vi "PCO_GetStorageStruct.vi"(8 "error in (no error)":errorcluster {"code" format="%x"}, 11 "ph":u64) -> (0 "error out":errorcluster {"code" format="%x"}, 1 "strStorage":T1, 2 "ErrorMessage":i32 format="%x", 3 "ph out":u64)   [LabVIEW 2019, in "SDK.lvlib" / "StorageControl.lvlib"]
doc: "<b>Description:</b>\nInformation about camera internal memory (CamRAM) is queried from the camera and the variables of the PCO_Storage structure are filled with this information. This function is a combined version of the functions, which request information about the current settings of storage related parameter. For a detailed description of each parameter see the functions in this chapter.\n\n<b>Supported camera type:</b>\npco.dimax, pco.1200, pco.1600, pco.2000, pco.4000\n\n<b>Descriptor dependency:</b>\ndwGeneralCapsDESC1: NO_RECORDER"
uses:
  StorageControl.lvlib
  Structures/Structures.lvlib
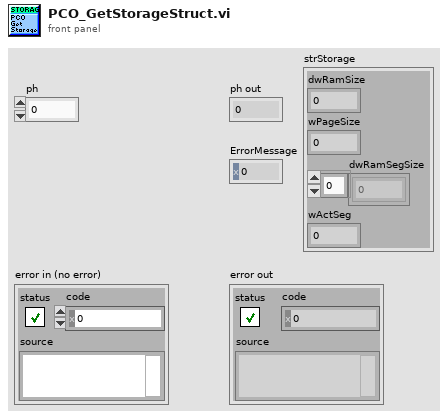
[diagram p1: front panel]
types:
  T1 = cluster{"dwRamSize":u32, "wPageSize":u16, "dwRamSegSize":u32[], "wActSeg":u16}
  T2 = cluster{"wSize":u16, "ZZwAlignDummy1":u16, "dwRamSize":u32, "wPageSize":u16, "ZZwAlignDummy4":u16, "dwRamSegSize":cluster{u32, u32, u32, u32}, "ZZdwDummyrs":cluster{u32, u32, u32, u32, u32, u32, u32, u32, u32, u32, u32, u32, u32, u32, u32, u32, u32, u32, u32, u32}, "wActSeg":u16, "ZZwDummy":cluster{u16, u16, u16, u16, u16, u16, u16, u16, u16, u16, u16, u16, u16, u16, u16, u16, u16, u16, u16, u16, u16, u16, u16, u16, u16, u16, u16, u16, u16, u16, u16, u16, u16, u16, u16, u16, u16, u16, u16}}
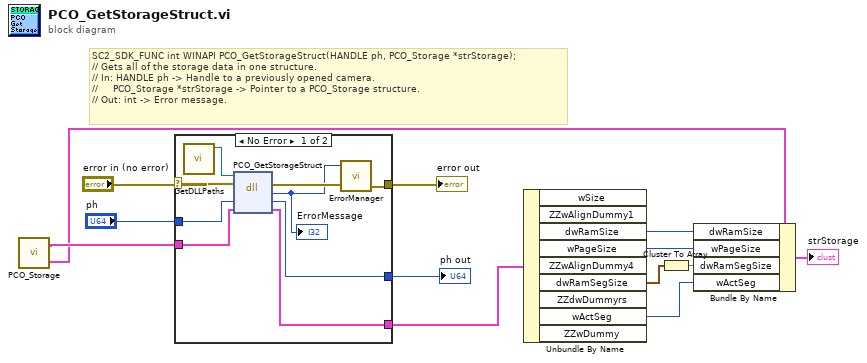
[diagram p0: block diagram]
diagram:
  # "SC2_SDK_FUNC int WINAPI PCO_GetStorageStruct(HANDLE ph, PCO_Storage *strStorage);\n// Gets all of the storage data in one structure.\n// In: HANDLE ph -> Handle to a previously opened camera.\n//     PCO_Storage *strStorage -> Pointer to a PCO_Storage structure.\n// Out: int -> Error message."
  n1 = call "PCO_Storage.vi"() -> ("PCO_Storage"=w7:T1, "PCO_Storage_Raw"=w9:T2)  [unwired: 4 in, 2 out]
  n2 = case shown="No Error" "error in (no error)" {
    selector: "error in (no error)" -> [w18 w25]
    tunnel: "ph" -> [w22 w24]
    tunnel: [w21 w24] -> w12
    tunnel: w9 -> [w20 w23]
    tunnel: [w19 w23] -> w8
    tunnel: [w16 w25] -> w11
    frame No Error {
      n3 = call "GetDLLPaths.vi"() -> ("SC2_Cam_Path"=w14:path)  [unwired: 9 in, 2 out]
      n4 = dll-call lib="?" fn="PCO_GetStorageStruct"(path in=w14, error in=w18, "ph"=w22, "strStorage"=w20) -> (error out=w17:errorcluster, "return type"=w15:i32, "ph"=w21:u64, "strStorage"=w19:T2)  [unwired: 1 in, 1 out]
      "ErrorMessage" <- w15
      n5 = call "ErrorManager.vi"("error in (no error)"=w17, "error code"=w15) -> ("error out"=w16:errorcluster)  [unwired: 3 in]
    }
    frame Error {
    }
  }
  "ph out" <- w12
  "error out" <- w11
  n6 = Unbundle By Name(w8) -> ("dwRamSize"=w6:u32, "wPageSize"=w5:u16, "dwRamSegSize"=w2:cluster{u32, u32, u32, u32}, "wActSeg"=w4:u16)  [unwired: 5 out]
  n7 = Cluster To Array(cluster=w2) -> (array=w3:u32[])
  n8 = Bundle By Name(cluster=w7, "dwRamSize"=w6, "wPageSize"=w5, "dwRamSegSize"=w3, "wActSeg"=w4) -> (→"strStorage":T1)
